vi "Randomize (test set).vi"(0 "Nr of test cases":i32, 1 "Nr or all cases":i32) -> (2 "Switch":i32[](array[numeric]), 3 "Indices (train)":i32[](array[numeric]), 4 "Indices (test)":i32[](array[numeric]))   [LabVIEW 2010]
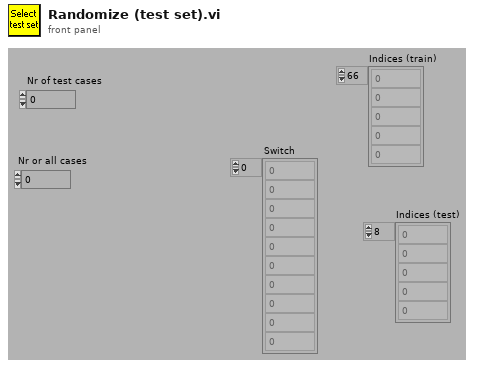
[diagram p1: front panel]
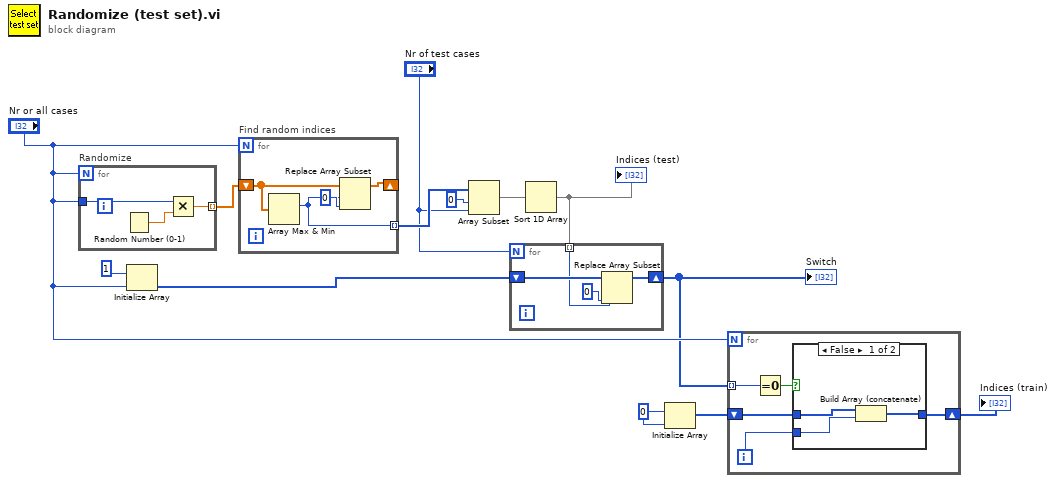
[diagram p0: block diagram]
diagram:
  w2 = 0 ("Element Data")
  n1 = for "Randomize" {
    N: "Nr or all cases" -> [_]
    tunnel: "Nr or all cases" -> [w16]
    tunnel: [w14] -> w9 mode=indexing
    n2 = Random Number (0-1)() -> (number: 0 to 1=w15:dbl)
    n3 = Multiply(x=w16, y=w15) -> (x*y=w14:dbl)
  }
  n4 = Initialize Array(1, "Nr or all cases") -> (w6:i32[])
  n5 = for "Find random indices" {
    N: "Nr or all cases" -> [_]
    shift-right: [w18] -> _
    shift-left: w9 -> [w19]
    tunnel: [w17] -> w12 mode=indexing
    n6 = Array Max & Min(array=w19) -> (max index (indices)=w17:i32)  [unwired: 3 out]
    n7 = Replace Array Subset(array=w19, new element=0 ("Array Index"), index=w17) -> (w18:dbl[])
  }
  n8 = Array Subset(array=w12, index=0 ("Array Index"), length="Nr of test cases") -> (w13:i32[])
  n9 = Sort 1D Array(array=w13) -> (sorted array=w7:i32[])
  "Indices (test)" <- w7
  n10 = for {
    N: "Nr of test cases" -> [_]
    tunnel: w7 -> [w21] mode=indexing
    shift-right: [w23] -> w4
    shift-left: w6 -> [w24]
    n11 = Replace Array Subset(array=w24, new element=0 ("Element Data"), index=w21) -> (w23:i32[])
  }
  "Switch" <- w4
  n12 = Initialize Array(w2, w2) -> (w3:i32[])
  n13 = for {
    N: "Nr or all cases" -> [_]
    tunnel: w4 -> [w29] mode=indexing
    shift-right: [w27] -> w1
    shift-left: w3 -> [w26]
    i -> [w25]
    n14 = Equal To 0?(x=w29) -> (x = 0?=w28:bool)
    n15 = case shown="False" w28 {
      tunnel: [w31 w33] -> w27
      tunnel: w26 -> [w32 w33]
      tunnel: w25 -> [w30 _]
      frame False {
        n16 = Build Array (concatenate)(w32, w30) -> (w31:i32[])
      }
      frame True {
      }
    }
  }
  "Indices (train)" <- w1
